vi "Receive.vi"(7 "Msg in":refnum<class "Msg Strategy.lvclass">, 11 "Destroy jettl State in":refnum<class "Destroy jettl State.lvclass">) -> (5 "Msg out":refnum<class "Msg Strategy.lvclass">)   [LabVIEW 2021, in "jettl.lvlib" / "Destroy jettl State.lvclass"]
uses:
  Destroy jettl State.lvclass
  Msg Strategy/Msg Strategy.lvclass
  Msgs/Last Ack/Last Ack Msg/Last Ack Msg.lvclass
  C:/git/jettl/src/jettl/Msg Strategy/Msg Strategy.lvclass
  Destroy jettl State.lvclass/Destroy jettl State.ctl
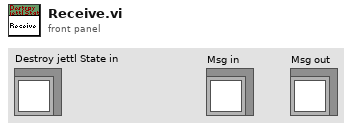
[diagram p1: front panel]
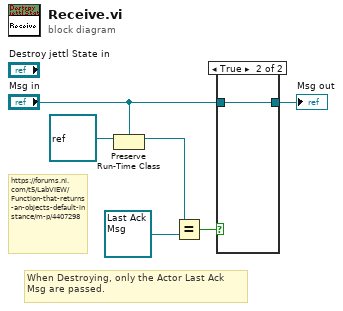
[diagram p0: block diagram]
diagram:
  # "https://forums.ni.com/t5/LabVIEW/Function-that-returns-an-objects-default-instance/m-p/4407298"
  # "When Destroying, only the Actor Last Ack Msg are passed."
  n1 = Preserve Run-Time Class(object in=refnum<class> refnum ("LabVIEW Object"), 2:"Msg in") -> (object out=w1:refnum<class "Msg Strategy.lvclass">)  [unwired: 1 in, 1 out]
  n2 = Equal?(x=w1, y=refnum<class "Last Ack Msg.lvclass"> refnum ("LVCAM Nest Destroyed.lvlib:LVCAM Nest Destroyed Msg.lvclass")) -> (x = y?=w5:bool)
  n3 = case shown="True" w5 {
    tunnel: [_ w7] -> w6
    tunnel: "Msg in" -> [_ w7]
    frame False {
    }
    frame True {
    }
  }
  "Msg out" <- w6
